vi "GetMatlabBoundControlCollection.vi"(11 "ExpID":string) -> (3 "Bound Controls":T1[](array[typedef]))   [LabVIEW 2017]
uses:
  Types/ControlValueChangeEventBindingType.ctl
  Types/MatlabBindingDirectionEnum.ctl
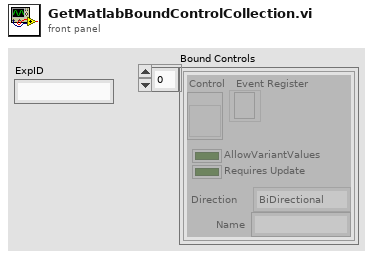
[diagram p1: front panel]
types:
  T1 = typedef "ControlValueChangeEventBindingType.ctl" = cluster{"Control":refnum<vi>, "Event Register":refnum<event-registration>, "AllowVariantValues":bool, "Direction":T2, "Requires Update":bool, "Name":string}
  T2 = typedef "MatlabBindingDirectionEnum.ctl" = enum16{"BiDirectional", "FromMatlab", "ToMatlab"}
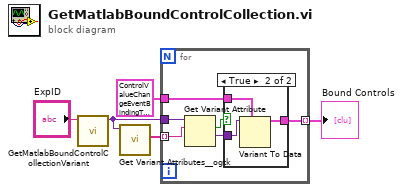
[diagram p0: block diagram]
diagram:
  n1 = call "GetMatlabBoundControlCollectionVariant.vi"("ExpID"="ExpID") -> ("BoundControlCollectionVariant"=w3:variant)  [unwired: 10 in]
  n2 = call <userlib>:"Get Variant Attributes__ogtk.vi"("Variant"=w3) -> ("names"=w4:string[])  [unwired: 3 in, 3 out]
  n3 = for {
    tunnel: w4 -> [w10] mode=indexing
    tunnel: w3 -> [w11]
    tunnel: T1 {"Control"=refnum, "Event Register"=refnum, "AllowVariantValues"=FALSE, "Direction"=enum."BiDirectional", "Requires Update"=FALSE, "Name"=""} -> [w9]
    tunnel: [w7] -> w1 mode=indexing
    n4 = Get Variant Attribute(Variant=w11, name=w10) -> (found=w6:bool, value=w8:variant)  [unwired: 2 in, 2 out]
    n5 = case shown="True" w6 {
      tunnel: w9 -> [w12 w15]
      tunnel: w8 -> [_ w14]
      tunnel: [w12 w13] -> w7
      frame False {
      }
      frame True {
        n6 = Variant To Data(type=w15, Variant=w14) -> (data=w13:T1)  [unwired: 1 in, 1 out]
      }
    }
  }
  "Bound Controls" <- w1
